vi "Mixer.Globals.vi"() -> ()   [LabVIEW 2020]
panel:
  in  "Height":i32=405
  in  "Width":i32=670
  out "ready":bool
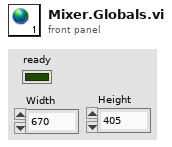
[diagram p1: front panel]
diagram:
